vi "New Config to Queue.vi"(8 "error in":errorcluster, 11 "queue in":T1) -> (0 "error out":errorcluster, 3 "queue out":T1)   [LabVIEW 2017, in "NI_LVConfig.lvlib"]
uses:
  <vilib>/Utility/config.llb/NI_LVConfig.lvlib
  <vilib>/Utility/config.llb/Config Queue.ctl
  <vilib>/Utility/config.llb/Config Data.ctl
  <vilib>/Utility/config.llb/Section.ctl
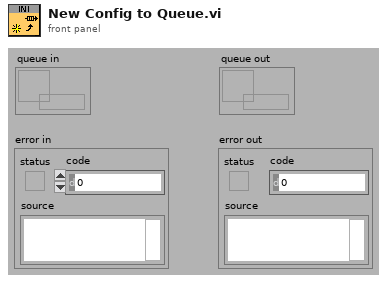
[diagram p1: front panel]
types:
  T1 = typedef "NI_LVConfig.lvlib/Config Queue.ctl" = refnum<queue>
  T2 = typedef "NI_LVConfig.lvlib/Section.ctl" = cluster{"name":string, "comment":string, "kvc":string[][]}
  T3 = typedef "NI_LVConfig.lvlib/Config Data.ctl" = cluster{"sections":T2[], "path":path, "dirty":bool}
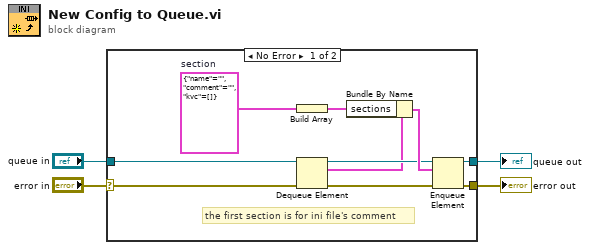
[diagram p0: block diagram]
diagram:
  n1 = case shown="No Error" "error in" {
    selector: "error in" -> [w6 w15]
    tunnel: [w14 w15] -> w4
    tunnel: [w12 w16] -> w3
    tunnel: "queue in" -> [w8 w16]
    frame No Error {
      w5 = T2 {"name"="", "comment"="", "kvc"=[]}  # section
      # "the first section is for ini file's comment"
      n2 = Build Array(w5) -> (w7:T2[])
      n3 = Dequeue Element(queue=w8, error in (no error)=w6) -> (queue out=w10:T1, element=w9:T3, error out=w13:errorcluster)  [unwired: 2 out]
      n4 = Bundle By Name(cluster=w9, "sections"=w7) -> (w11:T3)
      n5 = Enqueue Element(queue=w10, element=w11, error in (no error)=w13) -> (queue out=w12:T1, error out=w14:errorcluster)  [unwired: 2 out]
    }
    frame Error {
    }
  }
  "error out" <- w4
  "queue out" <- w3
